vi "Main.vi"() -> ()   [LabVIEW 2017]
doc: "The myRIO Project template acquires acceleration data from the onboard accelerometer and displays the changes of acceleration values in a waveform chart."
uses:
  Coords Input Cluster.ctl
  Motor Status Enum.ctl
  <vilib>/myRIO/Instrument Drivers/Onboard IO/PWM/typedefs/PWM Reference.ctl
  <vilib>/myRIO/Common/Instrument Driver Framework/Utilities/typedefs/myRIO Generic Hardware Reference.ctl
  <vilib>/myRIO/Common/Instrument Driver Framework/Utilities/typedefs/Hardware Version Enum.ctl
  <vilib>/myRIO/Common/Instrument Driver Framework/Utilities/typedefs/myRIO v1.0 Reference.ctl
  <vilib>/myRIO/Common/Instrument Driver Framework/Utilities/typedefs/Generic FPGA Reference.ctl
  <vilib>/myRIO/Common/Instrument Driver Framework/myRIO v1.0/PWM/typedefs/PWM Channels Enum.ctl
  <vilib>/myRIO/Instrument Drivers/Onboard IO/PWM/typedefs/PWM Configuration.ctl
  <vilib>/userdefined/High Color/nirio_resource_hc.ctl
  <vilib>/myRIO/Common/Instrument Driver Framework/Utilities/vis/Is FPGA Ref Available.vi
  <vilib>/myRIO/Common/Instrument Driver Framework/myRIO v1.0/PWM/vis/myRIO v1.1 Open PWM.vi
  <vilib>/myRIO/Instrument Drivers/Onboard IO/PWM/vis/Set Duty Cycle and Frequency.vi
  <vilib>/myRIO/Common/Instrument Driver Framework/Utilities/vis/Validate Channels.vi
  <vilib>/myRIO/Common/Instrument Driver Framework/myRIO v1.0/PWM/vis/myRIO v1.0 Reserve PWM.vi
  <vilib>/myRIO/Common/Instrument Driver Framework/myRIO v1.0/UART/vis/myRIO v1.0 Close UART.vi
  <vilib>/myRIO/Common/Instrument Driver Framework/myRIO v1.0/PWM/vis/myRIO v1.0 Build MUX Configuration PWM.vi
  <vilib>/myRIO/Common/Instrument Driver Framework/myRIO v1.0/Resource Manager/vis/myRIO v1.0 Reserve Channel List.vi
  <vilib>/myRIO/Common/Instrument Driver Framework/myRIO v1.0/Resource Manager/vis/myRIO v1.0 Create Configuration List.vi
  <vilib>/myRIO/Common/Instrument Driver Framework/myRIO v1.0/Resource Manager/vis/myRIO v1.0 Reserve Channel.vi
  <vilib>/myRIO/Common/Instrument Driver Framework/myRIO v1.0/Resource Manager/vis/myRIO v1.0 Unreserve Channel.vi
  <vilib>/myRIO/Common/Instrument Driver Framework/myRIO v1.0/Resource Manager/vis/myRIO v1.0 Build Mutex Name.vi
  <vilib>/Utility/VariantDataType/GetNumericInfo.vi
  <vilib>/Utility/error.llb/Error Cluster From Error Code.vi
  <vilib>/myRIO/Common/Instrument Driver Framework/myRIO v1.0/myRIO v1.1 Open.vi
  <vilib>/myRIO/Common/Instrument Driver Framework/Utilities/vis/IO Manager.vi
  <vilib>/myRIO/Common/Instrument Driver Framework/Utilities/vis/Configuration Manager.vi
  <vilib>/myRIO/Common/Instrument Driver Framework/myRIO v1.0/Resource Manager/vis/myRIO v1.0 Configure IO.vi
  <vilib>/myRIO/Common/Instrument Driver Framework/myRIO v1.0/myRIO v1.0 Close.vi
  <vilib>/myRIO/Common/Instrument Driver Framework/myRIO v1.0/PWM/vis/myRIO v1.0 Write PWM.vi
  <vilib>/myRIO/Common/Instrument Driver Framework/roboRIO v1.0/PWM/vis/roboRIO v1.0 Write PWM.vi
  <vilib>/myRIO/Common/Instrument Driver Framework/Utilities/vis/FPGA Ref Manager.vi
  <vilib>/myRIO/Common/Instrument Driver Framework/myRIO v1.0/myRIO v1.0 Reset FPGA.vi
  <vilib>/myRIO/Common/Instrument Driver Framework/myRIO v1.0/IRQ/vis/myRIO v1.0 IRQ Info FGV.vi
  <vilib>/myRIO/Common/Instrument Driver Framework/myRIO v1.0/IRQ/vis/myRIO v1.0 Timer IRQ Info FGV.vi
  <vilib>/myRIO/Express VI/Onboard IO/PWM/PWM Express VI.xnode
  <vilib>/myRIO/Instrument Drivers/Onboard IO/PWM/vis/myRIO PWM Open.xnode
  <vilib>/myRIO/Instrument Drivers/Utilities/Utilities.lvlib
  <vilib>/myRIO/Instrument Drivers/Onboard IO/PWM/PWM.lvlib
panel:
  out "Solenoid\nON/OFF":bool
  out "Kicker Outputs":T1
  in  "Kicker Inputs":T2
  out "Y Acceleration":dbl[][](graph)
  out "Y Displacment":dbl[][](graph)
  out "Y Velocity":dbl[][](graph)
  in  "Y Axis Setpoint":T3
  in  "Coordinates Input":T4={"X-axis (mm)"=0.0, "Y-axis (mm)"=0.0, "Y dist  target \nthreshold (mm)"=1.0, "X dist target\nthreshold (mm)"=0.0} {"X dist target\nthreshold (mm)" min=0.0; "Y dist  target \nthreshold (mm)" min=0.0}
  out "Y Axis":T5(graph)
  out "X Axis":T5(graph)
  in  "X Axis Setpoint":T6
  in  "stop":bool
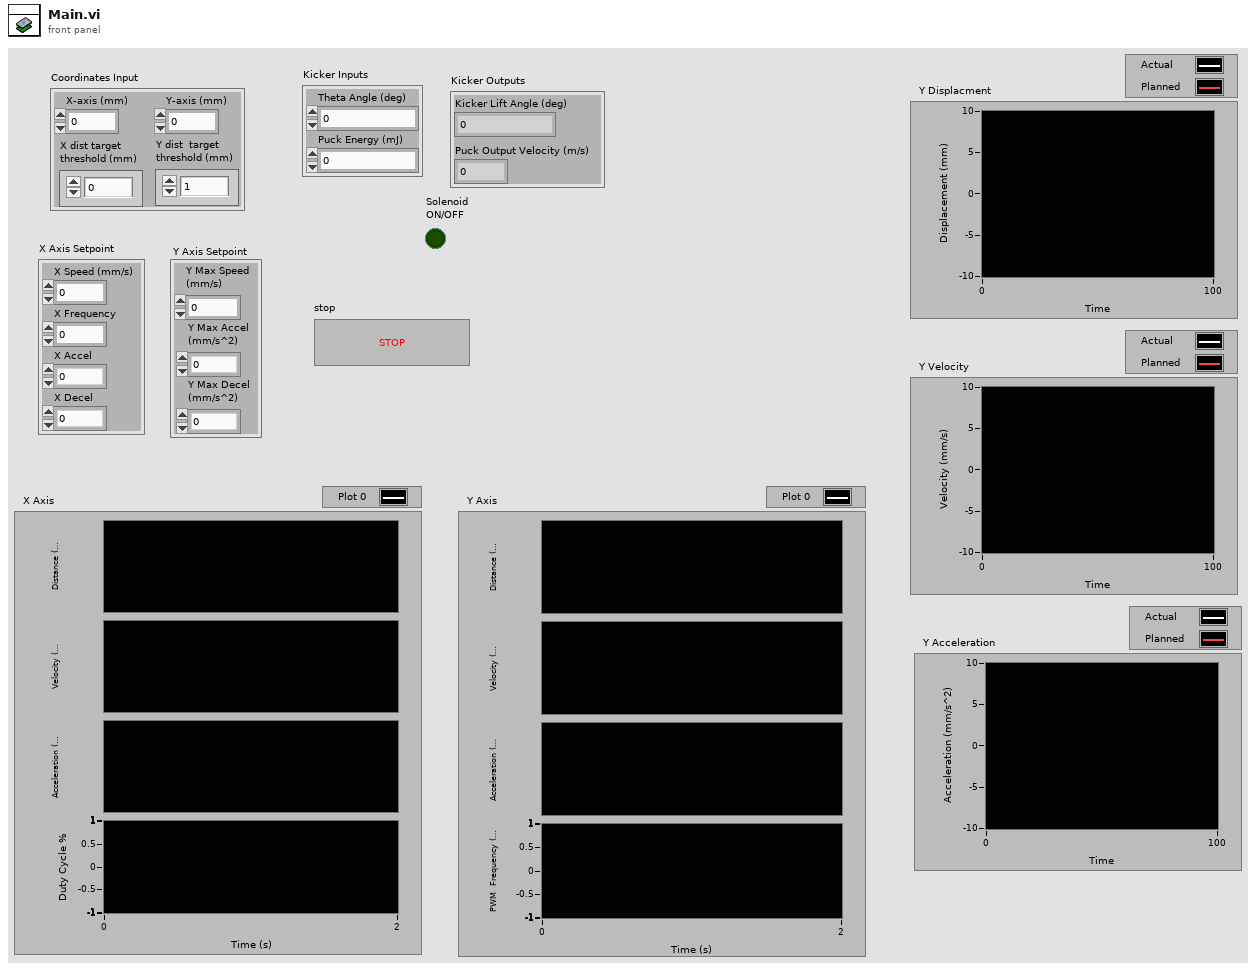
[diagram p1: front panel]
types:
  T1 = cluster{"Kicker Lift Angle (deg)":dbl, "Puck Output Velocity (m/s)":dbl}
  T2 = cluster{"Theta Angle (deg)":dbl, "Puck Energy (mJ)":dbl}
  T3 = cluster{"Y Max Speed \n(mm/s)":dbl, "Y Max Accel\n(mm/s^2)":dbl, "Y Max Decel \n(mm/s^2)":dbl}
  T4 = typedef "Coords Input Cluster.ctl" = cluster{"X-axis (mm)":dbl, "Y-axis (mm)":dbl, "Y dist  target \nthreshold (mm)":dbl, "X dist target\nthreshold (mm)":dbl}
  T5 = cluster{"X-axis distance":dbl, dbl, dbl, "X Frequency":dbl}
  T6 = cluster{"X Frequency":dbl, "X Accel":dbl, "X Decel":dbl, "X Speed (mm/s)":dbl}
  T7 = typedef "Motor Status Enum.ctl" = enum16{"Stop Motor", "Read Inputs", "Steady Speed", "Accelerate", "Decelerate"}
  T8 = cluster{"X Motor State":T7, "Y Motor State":T7, "X Axis Motor Params":cluster{"X Frequency":dbl, "X FWD/RVS":bool, "X Accel":dbl, "X Decel":dbl, "X Duty Cycle %":dbl}, "Telemetry":dbl[][], "stop":bool, "Y Axis Motor Params":cluster{"Y Frequency":dbl, "Y FWD/RVS":bool, "Y Accel":dbl, "Y Decel":dbl}}
  T9 = cluster{"Coordinates Input ":T4, "X Axis Setpoint":cluster{"X Frequency":dbl, "X Accel":dbl, "X Decel":dbl, "X Speed (mm/s)":dbl}, "Y Axis Setpoint":cluster{"Y Max Speed \n(mm/s)":dbl, "Y Max Accel\n(mm/s^2)":dbl, "Y Max Decel \n(mm/s^2)":dbl}}
  T10 = cluster{"Kicker Lift Angle (°)":dbl, "Puck Output Velocity (m/s)":dbl}
  T11 = cluster{"Y Velocity":dbl[][], "Y Displacment":dbl[][], "Y Acceleration":dbl[][]}
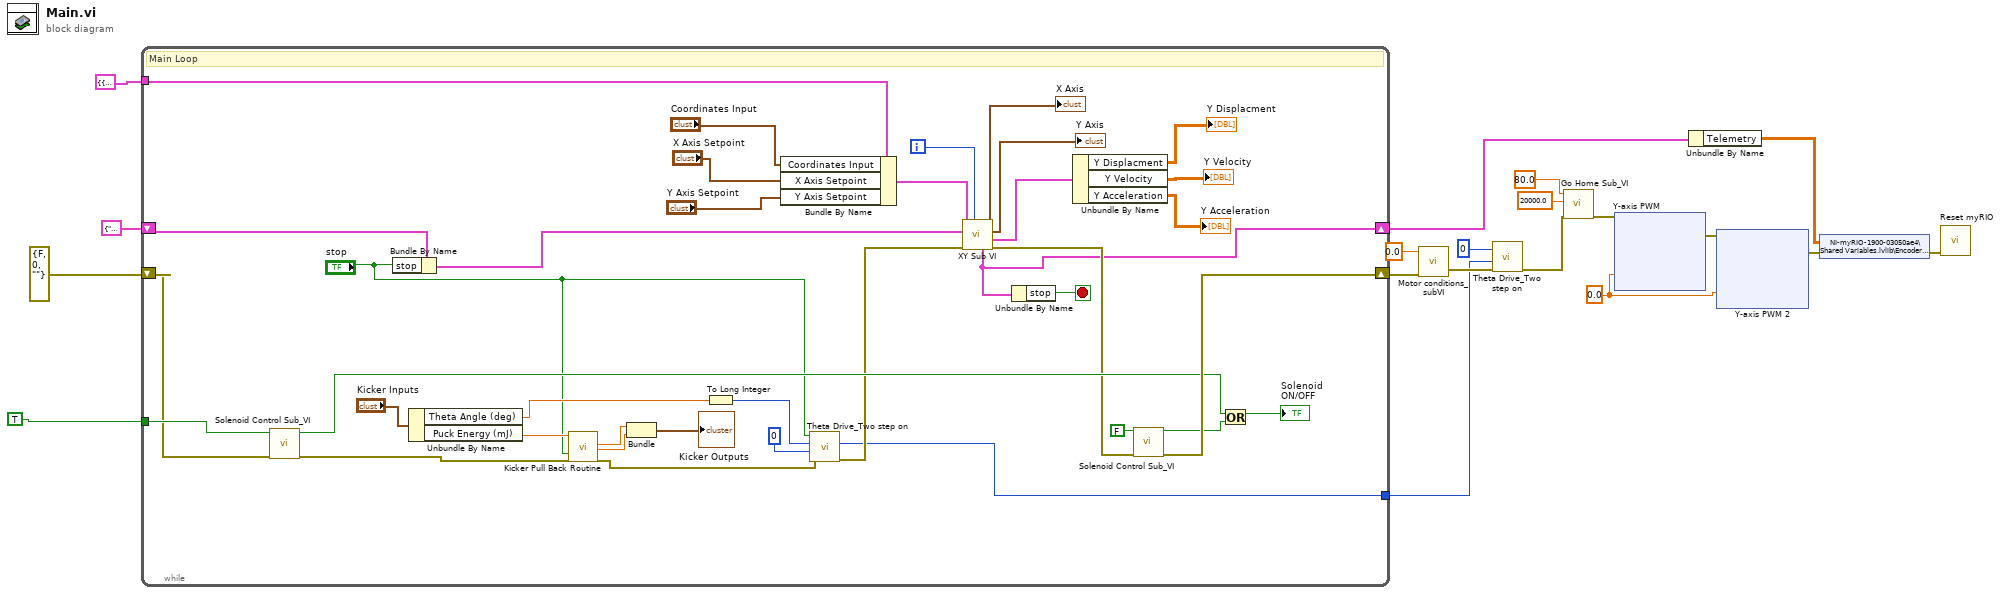
[diagram p0: block diagram]
diagram:
  w15 = 0.0 ("Frequency [Hz]")
  n1 = while {
    shift-right: [w52] -> w6
    shift-left: errorcluster {"status"=FALSE, "code"=0, "source"=""} ("error in (no error)") -> [w53]
    tunnel: TRUE ("SOLENOID ON/OFF") -> [w56]
    shift-right: [w33] -> w8
    shift-left: T8 {"X Motor State"=enum."Stop Motor", "Y Motor State"=enum."Stop Motor", "X Axis Motor Params"={"X Frequency"=0.0, "X FWD/RVS"=FALSE, "X Accel"=0.0, "X Decel"=0.0, "X Duty Cycle %"=0.0}, "Telemetry"=[], "stop"=FALSE, "Y Axis Motor Params"={"Y Frequency"=0.0, "Y FWD/RVS"=FALSE, "Y Accel"=0.0, "Y Decel"=0.0}} ("XY State Machine Out") -> [w35]
    tunnel: T9 {"Coordinates Input "={"X-axis (mm)"=0.0, "Y-axis (mm)"=0.0, "Y dist  target \nthreshold (mm)"=1.0, "X dist target\nthreshold (mm)"=0.0}, "X Axis Setpoint"={"X Frequency"=0.0, "X Accel"=0.0, "X Decel"=0.0, "X Speed (mm/s)"=0.0}, "Y Axis Setpoint"={"Y Max Speed \n(mm/s)"=0.0, "Y Max Accel\n(mm/s^2)"=0.0, "Y Max Decel \n(mm/s^2)"=0.0}} ("XY Params Input") -> [w45]
    tunnel: [w20] -> w1
    i -> [w48]
    stop <- w32 stop-if-true
    # "Main Loop"
    n2 = call "Solenoid Control Sub_VI.vi"("error in (no error)"=w53, "SOLENOID ON/OFF"=w56) -> ("error out"=w30:errorcluster, "ON/OFF"=w51:bool)  [unwired: 8 in]
    n3 = Bundle By Name(cluster=w35, "stop"="stop") -> (w34:T8)
    n4 = Unbundle By Name("Kicker Inputs") -> ("Theta Angle (deg)"=w23:dbl, "Puck Energy (mJ)"=w29:dbl)
    n5 = call "Kicker Pull Back Routine.vi"("Puck Energy Requirement (mJ)"=w29, "stop"="stop", "error in (no error)"=w30) -> ("Kicker Lift Angle (°)"=w28:dbl, "Puck Output Velocity (m/s)"=w27:dbl, "error out"=w26:errorcluster)  [unwired: 12 in, 2 out]
    n6 = Bundle("Kicker Lift Angle (°)"=w28, "Puck Output Velocity (m/s)"=w27) -> (→"Kicker Outputs":T10)  [unwired: 1 in]
    n7 = To Long Integer(number=w23) -> (32bit integer=w22:i32)
    n8 = Bundle By Name(cluster=w45, "Coordinates Input"="Coordinates Input", "X Axis Setpoint"="X Axis Setpoint", "Y Axis Setpoint"="Y Axis Setpoint") -> (w46:T9)
    n9 = call "Theta Drive_Two step on.vi"("error in (no error)"=w26, "Start Location Step (-90to90)"=0, "Target Step (-90to90)"=w22, "stop"="stop") -> ("error out"=w25:errorcluster, "Current Step (-90to90)"=w20:i32)  [unwired: 4 in, 2 out]
    n10 = call "XY Sub VI.vi"("Loop Count"=w48, "error in (no error)"=w25, "XY State Machine In"=w34, "XY Params Input"=w46) -> ("error out"=w47:errorcluster, "Y Path Display"=w39:T11, "Y Axis"=→"Y Axis":T5, "X Axis"=→"X Axis":T5, "XY State Machine Out"=w33:T8)  [unwired: 3 in]
    n11 = Unbundle By Name(w33) -> ("stop"=w32:bool)
    n12 = Unbundle By Name(w39) -> ("Y Displacment"=→"Y Displacment":dbl[][], "Y Velocity"=→"Y Velocity":dbl[][], "Y Acceleration"=→"Y Acceleration":dbl[][])
    n13 = call "Solenoid Control Sub_VI.vi"("error in (no error)"=w47, "SOLENOID ON/OFF"=FALSE) -> ("error out"=w52:errorcluster, "ON/OFF"=w49:bool)  [unwired: 8 in]
    n14 = Or(x=w51, y=w49) -> (x .or. y?=→"Solenoid\nON/OFF":bool)
  }
  n15 = call "Motor conditions_subVI.vi"("Target Angle (°)"=0.0, "error in (no error)"=w6) -> ("error out"=w4:errorcluster)  [unwired: 11 in, 2 out]
  n16 = call "Theta Drive_Two step on.vi"("error in (no error)"=w4, "Start Location Step (-90to90)"=w1, "Target Step (-90to90)"=0) -> ("error out"=w3:errorcluster)  [unwired: 5 in, 3 out]
  n17 = call "Go Home Sub_VI.vi"("error in (no error)"=w3, "Homing Freq"=20000.0, "Homing Duty %"=80.0) -> ("error out"=w14:errorcluster)  [unwired: 7 in, 1 out]
  n18 = xnode "Y-axis PWM"("Frequency [Hz]"=w15, "error in (no error)"=w14) -> ("error out"=w17:errorcluster)
  n19 = Unbundle By Name(w8) -> ("Telemetry"=w7:dbl[][])
  n20 = xnode "Y-axis PWM 2"("Frequency [Hz]"=w15, "error in (no error)"=w17) -> ("error out"=w16:errorcluster)
  n21 = shared-variable "NI-myRIO-1900-03050ae4\\Shared Variables.lvlib\\Encoder Data"(w7, error in=w16) -> (error out=w18:errorcluster)
  n22 = call <vilib>:"Reset myRIO.vi"("error in (no error)"=w18) -> ()  [unwired: 10 in, 1 out]
